vi "JPL Auto Complex.vi"   [LabVIEW 2015]
types:
  T1 = cluster{"L Upper Value":dbl, "L Upper Max Speed":dbl, "L Actual Speed":dbl, "L Slowdown":dbl, "L Lower Value":dbl, "Limit Switches":bool, "Limit Switches":bool, "L Lower Max Speed":dbl}
  T2 = cluster{"Arm Angle Ref":dbl, "Arm Offset":dbl, bool}
  T3 = cluster{"R Upper Value":dbl, "R Upper Max Speed":dbl, "R Actual Speed":dbl, "R Slowdown":dbl, "R Lower Value":dbl, "Limit Switches":bool, "Limit Switches":bool, "R Lower Max Speed":dbl}
  T4 = cluster{"Arm Upper Speed Limit":dbl, "Arm Low Speed Limit":dbl}
  T5 = cluster{"Encoder Alarm Status":string, "Encoder Distance":dbl, "Encoder Direction":string, "Encoder Rate (distance/sec)":dbl}
  T6 = cluster{"Arm Angle":dbl, "Arm Difference (PID Input)":dbl}
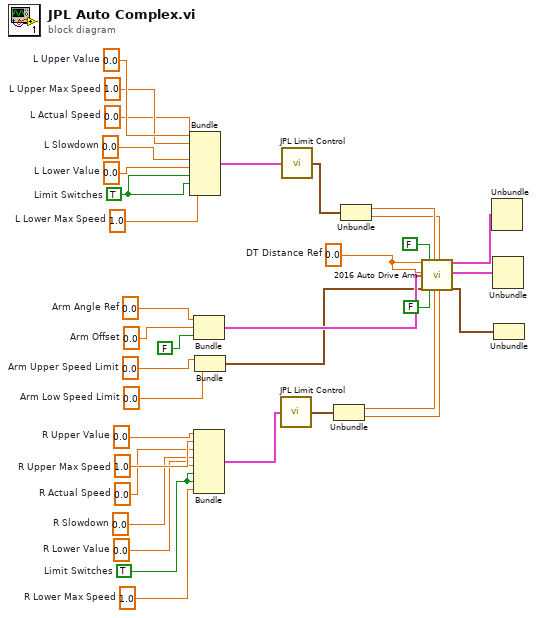
[diagram p0: block diagram]
diagram:
  w3 = 0.0  # R Lower Value
  w4 = 0.0  # R Slowdown
  w5 = 0.0  # R Actual Speed
  w1 = 1.0  # R Lower Max Speed
  w2 = TRUE  # Limit Switches
  w6 = 1.0  # R Upper Max Speed
  w7 = 0.0  # R Upper Value
  w8 = 0.0  # L Lower Value
  w9 = 0.0  # L Slowdown
  w10 = 0.0  # L Actual Speed
  w11 = 1.0  # L Lower Max Speed
  w12 = TRUE  # Limit Switches
  w13 = 1.0  # L Upper Max Speed
  w14 = 0.0  # L Upper Value
  w16 = 0.0  # Arm Low Speed Limit
  w17 = 0.0  # Arm Upper Speed Limit
  w19 = 0.0  # Arm Offset
  w20 = 0.0  # Arm Angle Ref
  w24 = 0.0  # DT Distance Ref
  n1 = Bundle("L Upper Value"=w14, "L Upper Max Speed"=w13, "L Actual Speed"=w10, "L Slowdown"=w9, "L Lower Value"=w8, "Limit Switches"=w12, "Limit Switches"=w12, "L Lower Max Speed"=w11) -> (w34:T1)  [unwired: 1 in]
  n2 = Bundle("Arm Angle Ref"=w20, "Arm Offset"=w19, FALSE) -> (w22:T2)  [unwired: 1 in]
  n3 = Bundle("R Upper Value"=w7, "R Upper Max Speed"=w6, "R Actual Speed"=w5, "R Slowdown"=w4, "R Lower Value"=w3, "Limit Switches"=w2, "Limit Switches"=w2, "R Lower Max Speed"=w1) -> (w15:T3)  [unwired: 1 in]
  n4 = Bundle("Arm Upper Speed Limit"=w17, "Arm Low Speed Limit"=w16) -> (w21:T4)  [unwired: 1 in]
  n5 = call "JPL Limit Control.vi"("Limit Inputs"=w15) -> ("Limit Output"=w31:cluster{"Positive Out":dbl, "Negative Out":dbl})  [unwired: 4 in]
  n6 = call "JPL Limit Control.vi"("Limit Inputs"=w34) -> ("Limit Output"=w35:cluster{"Positive Out":dbl, "Negative Out":dbl})  [unwired: 4 in]
  n7 = Unbundle(w31) -> ("Positive Out"=w30:dbl, "Negative Out"=w29:dbl)
  n8 = Unbundle(w35) -> ("Positive Out"=w33:dbl, "Negative Out"=w32:dbl)
  n9 = call "2016 Auto Drive Arm.vi"("Left Side Speed"=w24, "Right Side Speed"=w24, "Arm Reference"=w22, "Arm Limits"=w21, "Left Side Reset"=FALSE, "Right Side Reset"=FALSE, "Left Upper Limit"=w33, "Right Upper Limit"=w30, "Left Lower Limit"=w32, "Right Lower Limit"=w29) -> ("Encoder Status"=w28:T5, "Encoder Status 2"=w27:T5, "Arm Data"=w23:T6)  [unwired: 7 in]
  n10 = Unbundle(w28) -> ()  [unwired: 4 out]
  n11 = Unbundle(w27) -> ()  [unwired: 4 out]
  n12 = Unbundle(w23) -> ()  [unwired: 2 out]
